vi "Sousvi1.vi"(2 "Array":bool[](array[boolean]), 3 "Coffee extraction":bool) -> (0 "appended array":string[][](array[string]), 1 "Nombre de colonnes":i32)   [LabVIEW 2022 SP3]
panel:
  out "?":string
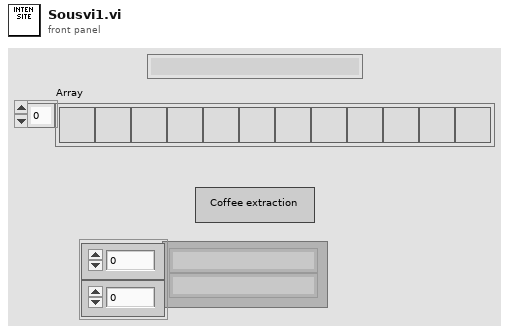
[diagram p1: front panel]
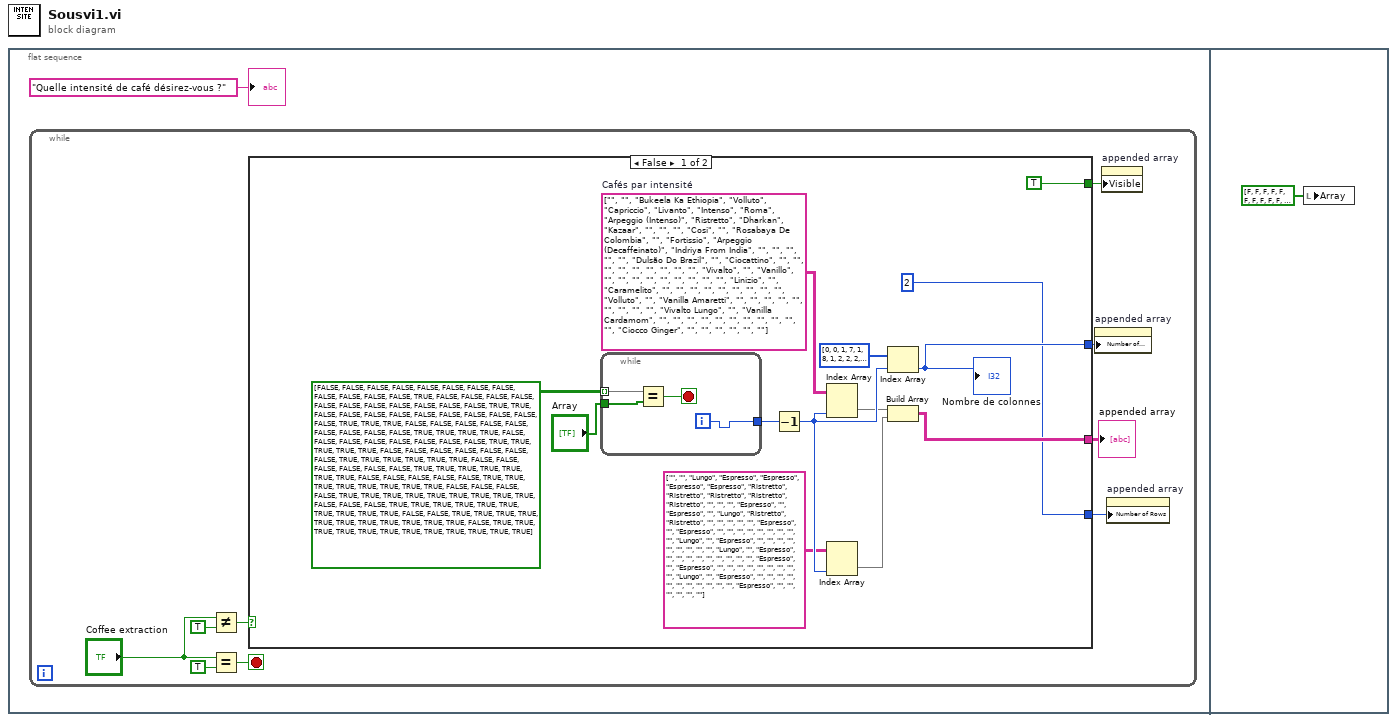
[diagram p0: block diagram]
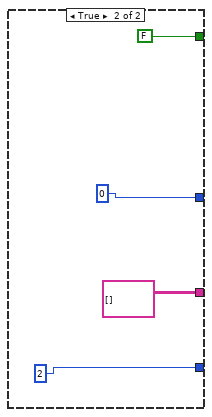
[diagram p2: hidden frame]
diagram:
  n1 = flat-sequence {
    frame #0 {
      n2 = while {
        stop <- w9 stop-if-true
        n3 = Not Equal?(x="Coffee extraction", y=TRUE) -> (x != y?=w7:bool)
        n4 = Equal?(x="Coffee extraction", y=TRUE) -> (x = y?=w9:bool)
        n5 = case shown="False" w7 {
          tunnel: [TRUE FALSE] -> w5
          tunnel: [w13 string[][] []] -> w4
          tunnel: [w12 0] -> w3
          tunnel: [2 2] -> w2
          frame False {
            w15 = string[][] [["", "", "Bukeela Ka Ethiopia", "Volluto", "Capriccio", "Livanto", "Intenso", "Roma", "Arpeggio (Intenso)", "Ristretto", "Dharkan", "Kazaar"], ["", "", "", "Cosi", "", "Rosabaya De Colombia", "", "Fortissio", "Arpeggio (Decaffeinato)", "Indriya From India", "", ""], ["", "", "", "Dulsão Do Brazil", "", "Ciocattino", "", "", "", "", "", ""], ["", "", "", "Vivalto", "", "Vanillo", "", "", "", "", "", ""], ["", "", "", "Linizio", "", "Caramelito", "", "", "", "", "", ""], ["", "", "", "Volluto", "", "Vanilla Amaretti", "", "", "", "", "", ""], ["", "", "", "Vivalto Lungo", "", "Vanilla Cardamom", "", "", "", "", "", ""], ["", "", "", "", "", "Ciocco Ginger", "", "", "", "", "", ""]]  # Cafés par intensité
            n6 = while {
              tunnel: bool[][] [[FALSE, FALSE, FALSE, FALSE, FALSE, FALSE, FALSE, FALSE, FALSE, FALSE, FALSE, FALSE], [TRUE, FALSE, FALSE, FALSE, FALSE, FALSE, FALSE, FALSE, FALSE, FALSE, FALSE, FALSE], [TRUE, TRUE, FALSE, FALSE, FALSE, FALSE, FALSE, FALSE, FALSE, FALSE, FALSE, FALSE], [TRUE, TRUE, TRUE, FALSE, FALSE, FALSE, FALSE, FALSE, FALSE, FALSE, FALSE, FALSE], [TRUE, TRUE, TRUE, TRUE, FALSE, FALSE, FALSE, FALSE, FALSE, FALSE, FALSE, FALSE], [TRUE, TRUE, TRUE, TRUE, TRUE, FALSE, FALSE, FALSE, FALSE, FALSE, FALSE, FALSE], [TRUE, TRUE, TRUE, TRUE, TRUE, TRUE, FALSE, FALSE, FALSE, FALSE, FALSE, FALSE], [TRUE, TRUE, TRUE, TRUE, TRUE, TRUE, TRUE, FALSE, FALSE, FALSE, FALSE, FALSE], [TRUE, TRUE, TRUE, TRUE, TRUE, TRUE, TRUE, TRUE, FALSE, FALSE, FALSE, FALSE], [TRUE, TRUE, TRUE, TRUE, TRUE, TRUE, TRUE, TRUE, TRUE, FALSE, FALSE, FALSE], [TRUE, TRUE, TRUE, TRUE, TRUE, TRUE, TRUE, TRUE, TRUE, TRUE, FALSE, FALSE], [TRUE, TRUE, TRUE, TRUE, TRUE, TRUE, TRUE, TRUE, TRUE, TRUE, TRUE, FALSE], [TRUE, TRUE, TRUE, TRUE, TRUE, TRUE, TRUE, TRUE, TRUE, TRUE, TRUE, TRUE]] -> [w27] mode=indexing
              tunnel: "Array" -> [w26]
              tunnel: [w24] -> w22
              i -> [w24]
              stop <- w25 stop-if-true
              n7 = Equal?(x=w27, y=w26) -> (x = y?=w25:bool)
            }
            n8 = Decrement(x=w22) -> (x-1=w21:i32)
            n9 = Index Array(array=w15, index (col)=w21) -> (element=w19:string[])  [unwired: 1 in]
            n10 = Index Array(array=string[][] [["", "", "Lungo", "Espresso", "Espresso", "Espresso", "Espresso", "Ristretto", "Ristretto", "Ristretto", "Ristretto", "Ristretto"], ["", "", "", "Espresso", "", "Espresso", "", "Lungo", "Ristretto", "Ristretto", "", ""], ["", "", "", "Espresso", "", "Espresso", "", "", "", "", "", ""], ["", "", "", "Lungo", "", "Espresso", "", "", "", "", "", ""], ["", "", "", "Lungo", "", "Espresso", "", "", "", "", "", ""], ["", "", "", "Espresso", "", "Espresso", "", "", "", "", "", ""], ["", "", "", "Lungo", "", "Espresso", "", "", "", "", "", ""], ["", "", "", "", "", "Espresso", "", "", "", "", "", ""]], index (col)=w21) -> (element=w20:string[])  [unwired: 1 in]
            n11 = Index Array(array=i32[] [0, 0, 1, 7, 1, 8, 1, 2, 2, 2, 1, 1], index=w21) -> (element=w12:i32)
            "Nombre de colonnes" <- w12
            n12 = Build Array(w19, w20) -> (w13:string[][])
          }
          frame True {
          }
        }
        "appended array" <- w4
        n13 = property on="appended array" class="Arr (strict)"("Number of Columns"=w3) -> ()  [unwired: 2 in, 2 out]
        n14 = property on="appended array" class="Arr (strict)"("Visible"=w5) -> ()  [unwired: 2 in, 2 out]
        n15 = property on="appended array" class="Arr (strict)"("Number of Rows"=w2) -> ()  [unwired: 2 in, 2 out]
      }
      "?" <- "Quelle intensité de café désirez-vous ?"
    }
    frame #1 {
      n16 = local write "Array"(bool[] [FALSE, FALSE, FALSE, FALSE, FALSE, FALSE, FALSE, FALSE, FALSE, FALSE, FALSE, FALSE] ("Array")) -> ()
    }
  }
